vi "01-Init.vi"() -> ()   [LabVIEW 2022 SP3, in "LV_VGS.lvlib"]
uses:
  LV_VGS.lvlib
  RemoteControlClient/VGS_RemoteControlClient.lvclass
panel:
  out "LastWarning":string
  out "LastError":string
  out "LastError":string
  out "Running,,,":i32
  in  "stop":bool
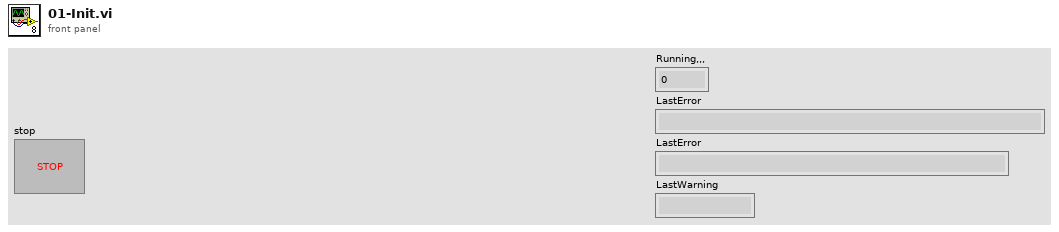
[diagram p1: front panel]
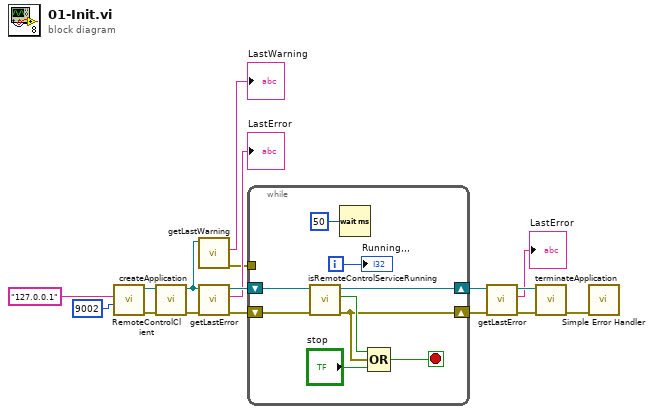
[diagram p0: block diagram]
diagram:
  n1 = call "RemoteControlClient.vi"("servicePort (9002)"=9002, "(localhost)"="127.0.0.1") -> ("error out"=w16:errorcluster, "VGS_RemoteControlClient out"=w17:refnum<class "VGS_RemoteControlClient.lvclass">)  [unwired: 8 in]
  n2 = call "createApplication.vi"("error in (no error)"=w16, "VGS_RemoteControlClient in"=w17) -> ("error out"=w9:errorcluster, "VGS_RemoteControlClient out"=w6:refnum<class "VGS_RemoteControlClient.lvclass">)  [unwired: 8 in]
  n3 = call "getLastWarning.vi"("VGS_RemoteControlClient in"=w6) -> ("error out"=w5:errorcluster, "LastWarning"=→"LastWarning":string)  [unwired: 8 in, 1 out]
  n4 = call "getLastError.vi"("error in (no error)"=w9, "VGS_RemoteControlClient in"=w6) -> ("error out"=w8:errorcluster, "LastError"=→"LastError":string, "VGS_RemoteControlClient out"=w10:refnum<class "VGS_RemoteControlClient.lvclass">)  [unwired: 7 in]
  n5 = while {
    shift-right: [w23] -> w2
    shift-left: w10 -> [w26]
    shift-right: [w19] -> w1
    shift-left: w8 -> [w22]
    tunnel: w5 -> [_]
    i -> [w21]
    stop <- w20 stop-if-true
    n6 = call "isRemoteControlServiceRunning.vi"("error in (no error)"=w22, "VGS_RemoteControlClient in"=w26) -> ("error out"=w19:errorcluster, "isRemoteControlServiceRunning"=w25:bool, "VGS_RemoteControlClient out"=w23:refnum<class "VGS_RemoteControlClient.lvclass">)  [unwired: 7 in]
    n7 = Wait (ms)(milliseconds to wait=u32 50) -> ()  [unwired: 1 out]
    n8 = Compound Arithmetic op=OR(w25, w19, "stop") -> (w20:bool)
    "Running,,," <- w21
  }
  n9 = call "getLastError.vi"("error in (no error)"=w1, "VGS_RemoteControlClient in"=w2) -> ("error out"=w11:errorcluster, "LastError"=→"LastError":string, "VGS_RemoteControlClient out"=w13:refnum<class "VGS_RemoteControlClient.lvclass">)  [unwired: 7 in]
  n10 = call "terminateApplication.vi"("error in (no error)"=w11, "VGS_RemoteControlClient in"=w13) -> ("error out"=w15:errorcluster)  [unwired: 8 in, 1 out]
  n11 = call <vilib>:"Simple Error Handler.vi"("error in (no error)"=w15) -> ()  [unwired: 4 in, 5 out]
